vi "Convex Polygon Intersection.vi"(8 "Y 2":dbl[](array[numeric]), 9 "X 2":dbl[](array[numeric]), 10 "Y 1":dbl[](array[numeric]), 11 "X 1":dbl[](array[numeric])) -> (0 "error":i32, 2 "Intersection Y":dbl[](array[numeric]), 3 "Intersection X":dbl[](array[numeric]))   [LabVIEW 2020, in "NI_AAL_Geometry.lvlib"]
doc: "Computes the intersection of two convex polygons."
uses:
  <vilib>/Analysis/NI_AAL_Geometry.lvlib
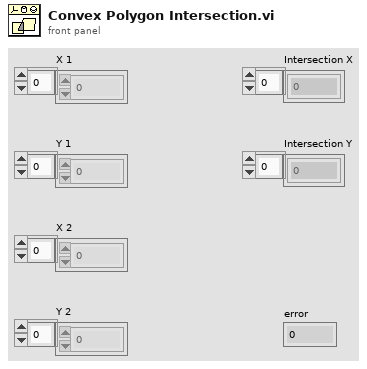
[diagram p1: front panel]
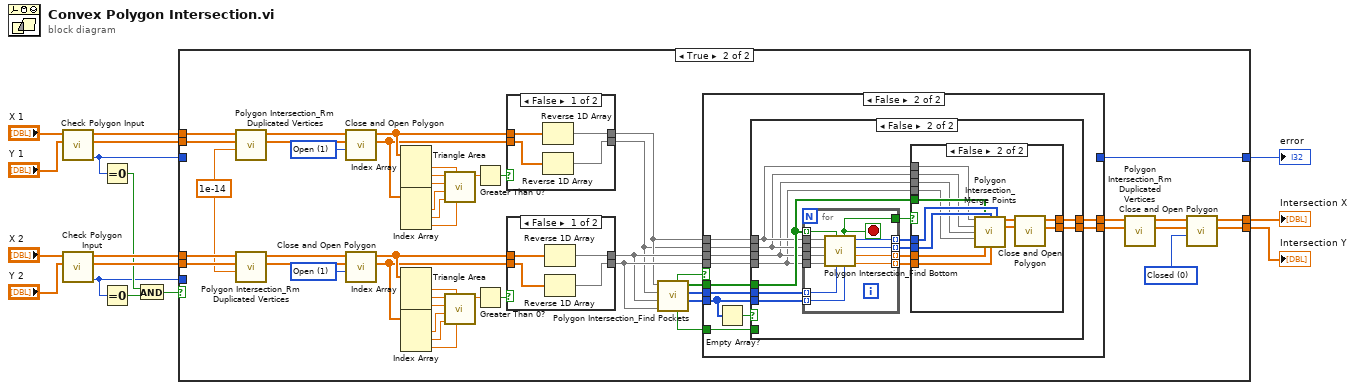
[diagram p0: block diagram]
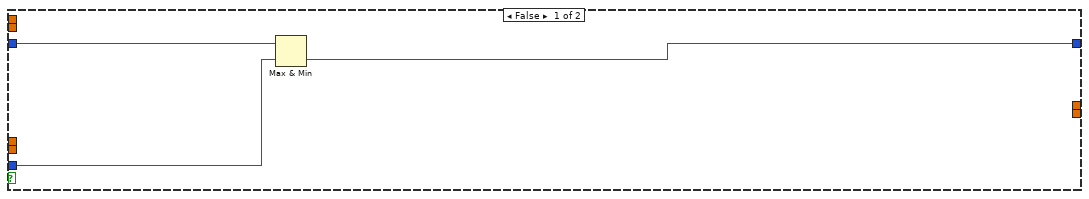
[diagram p2: hidden frame]
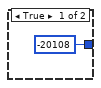
[diagram p3: hidden frame]
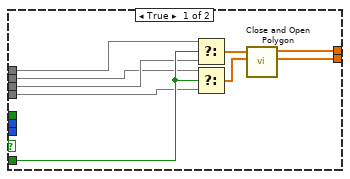
[diagram p4: hidden frame]
diagram:
  n1 = call <vilib>:"Check Polygon Input.vi"("Y In"="Y 1", "X In"="X 1") -> ("error"=w5:i32, "Y Out"=w12:dbl[], "X Out"=w13:dbl[])  [unwired: 7 in]
  n2 = call <vilib>:"Check Polygon Input.vi"("Y In"="Y 2", "X In"="X 2") -> ("error"=w4:i32, "Y Out"=w9:dbl[], "X Out"=w11:dbl[])  [unwired: 7 in]
  n3 = Equal To 0?(x=w5) -> (x = 0?=w8:bool)
  n4 = Equal To 0?(x=w4) -> (x = 0?=w7:bool)
  n5 = And(x=w8, y=w7) -> (x .and. y?=w6:bool)
  n6 = case shown="True" w6 {
    tunnel: w13 -> [_ w28]
    tunnel: w12 -> [_ w27]
    tunnel: w11 -> [_ w24]
    tunnel: w9 -> [_ w23]
    tunnel: w5 -> [w19 _]
    tunnel: w4 -> [w18 _]
    tunnel: [_ w30] -> w3
    tunnel: [w17 w50] -> w2
    tunnel: [_ w29] -> w1
    frame False {
      n7 = Max & Min(x=w19, y=w18) -> (min(x,y)=w17:i32)  [unwired: 1 out]
    }
    frame True {
      w20 = 1e-14 ("tolerance")
      w33 = u16 0 items=["Closed", "Open"] ("type")
      w64 = u16 1 items=["Closed", "Open"] ("type")
      w65 = u16 1 items=["Closed", "Open"] ("type")
      n8 = call <vilib>:"Polygon Intersection_Rm Duplicated Vertices.vi"("tolerance"=w20, "Y"=w27, "X"=w28) -> ("Y out"=w26:dbl[], "X out"=w25:dbl[])  [unwired: 7 in]
      n9 = call <vilib>:"Polygon Intersection_Rm Duplicated Vertices.vi"("tolerance"=w20, "Y"=w23, "X"=w24) -> ("Y out"=w22:dbl[], "X out"=w21:dbl[])  [unwired: 7 in]
      n10 = call <vilib>:"Close and Open Polygon.vi"("type"=w65, "Y In"=w26, "X In"=w25) -> ("Y Out"=w62:dbl[], "X Out"=w63:dbl[])  [unwired: 7 in]
      n11 = call <vilib>:"Close and Open Polygon.vi"("type"=w64, "Y In"=w22, "X In"=w21) -> ("Y Out"=w56:dbl[], "X Out"=w61:dbl[])  [unwired: 7 in]
      n12 = Index Array(array=w63) -> (element #1=w49:dbl, element #2=w48:dbl, element #3=w47:dbl)  [unwired: 3 in]
      n13 = Index Array(array=w62) -> (element #1=w46:dbl, element #2=w45:dbl, element #3=w44:dbl)  [unwired: 3 in]
      n14 = Index Array(array=w61) -> (element #1=w43:dbl, element #2=w42:dbl, element #3=w41:dbl)  [unwired: 3 in]
      n15 = Index Array(array=w56) -> (element #1=w40:dbl, element #2=w39:dbl, element #3=w38:dbl)  [unwired: 3 in]
      n16 = call <vilib>:"Triangle Area.vi"("y 3"=w44, "x 1"=w49, "y 2"=w45, "y 1"=w46, "x 3"=w47, "x 2"=w48) -> ("area"=w37:dbl)  [unwired: 5 in]
      n17 = call <vilib>:"Triangle Area.vi"("y 3"=w38, "x 1"=w43, "y 2"=w39, "y 1"=w40, "x 3"=w41, "x 2"=w42) -> ("area"=w35:dbl)  [unwired: 5 in]
      n18 = Greater Than 0?(x=w37) -> (x > 0?=w36:bool)
      n19 = Greater Than 0?(x=w35) -> (x > 0?=w34:bool)
      n20 = case shown="False" w36 {
        tunnel: w62 -> [w135 w138]
        tunnel: w63 -> [w137 w139]
        tunnel: [w136 w139] -> w52
        tunnel: [w134 w138] -> w51
        frame False {
          n21 = Reverse 1D Array(array=w137) -> (reversed array=w136:dbl[])
          n22 = Reverse 1D Array(array=w135) -> (reversed array=w134:dbl[])
        }
        frame True {
        }
      }
      n23 = case shown="False" w34 {
        tunnel: w56 -> [w129 w132]
        tunnel: w61 -> [w131 w133]
        tunnel: [w130 w133] -> w57
        tunnel: [w128 w132] -> w60
        frame False {
          n24 = Reverse 1D Array(array=w131) -> (reversed array=w130:dbl[])
          n25 = Reverse 1D Array(array=w129) -> (reversed array=w128:dbl[])
        }
        frame True {
        }
      }
      n26 = call <vilib>:"Polygon Intersection_Find Pockets.vi"("y2"=w60, "x2"=w57, "y1"=w51, "x1"=w52) -> ("index2"=w59:i32[], "index1"=w67:i32[], "left turn?"=w66:bool[], "inner?"=w58:bool, "complex or concave?"=w53:bool)  [unwired: 3 in]
      n27 = case shown="False" w53 {
        tunnel: w67 -> [_ w79]
        tunnel: w59 -> [_ w71]
        tunnel: w66 -> [_ w78]
        tunnel: [_ w77] -> w55
        tunnel: w52 -> [_ w76]
        tunnel: w51 -> [_ w75]
        tunnel: w57 -> [_ w74]
        tunnel: w60 -> [_ w73]
        tunnel: [_ w72] -> w54
        tunnel: w58 -> [_ w69]
        tunnel: [-20108 _] -> w50
        frame True {
        }
        frame False {
          n28 = Empty Array?(array=w71) -> (empty?=w70:bool)
          n29 = case shown="False" w70 {
            tunnel: w79 -> [_ w102]
            tunnel: w71 -> [_ w101]
            tunnel: w78 -> [_ w93]
            tunnel: [w81 w96] -> w77
            tunnel: [w80 w95] -> w72
            tunnel: w76 -> [w88 w92]
            tunnel: w75 -> [w85 w91]
            tunnel: w74 -> [w86 w90]
            tunnel: w73 -> [w84 w89]
            tunnel: w69 -> [w87 _]
            frame True {
              n30 = Select(t=w88, s=w87, f=w86) -> (s? t:f=w83:dbl[])
              n31 = Select(t=w85, s=w87, f=w84) -> (s? t:f=w82:dbl[])
              n32 = call <vilib>:"Close and Open Polygon.vi"("Y In"=w82, "X In"=w83) -> ("Y Out"=w80:dbl[], "X Out"=w81:dbl[])  [unwired: 8 in]
            }
            frame False {
              n33 = for {
                tunnel: w92 -> [w124]
                tunnel: w91 -> [w123]
                tunnel: w90 -> [w122]
                tunnel: w89 -> [w121]
                tunnel: w93 -> [w125] mode=indexing
                tunnel: w102 -> [w127] mode=indexing
                tunnel: w101 -> [w126] mode=indexing
                tunnel: [w118] -> w100 mode=indexing
                tunnel: [w117] -> w99 mode=indexing
                tunnel: [w120] -> w98 mode=indexing
                tunnel: [w119] -> w97 mode=indexing
                tunnel: [w116] -> w94
                stop <- w116 stop-if-true
                n34 = call <vilib>:"Polygon Intersection_Find Bottom.vi"("index2"=w126, "index1"=w127, "Left Turn?"=w125, "y2"=w121, "x2"=w122, "y1"=w123, "x1"=w124) -> ("y"=w119:dbl, "x"=w120:dbl, "index2 out"=w117:i32, "index1 out"=w118:i32, "isolate?"=w116:bool)
              }
              n35 = case shown="False" w94 {
                tunnel: w100 -> [_ w115]
                tunnel: w99 -> [_ w114]
                tunnel: w93 -> [_ w113]
                tunnel: w98 -> [_ w112]
                tunnel: w97 -> [_ w111]
                tunnel: [_ w104] -> w96
                tunnel: [_ w103] -> w95
                tunnel: w90 -> [_ w110]
                tunnel: w89 -> [_ w109]
                tunnel: w92 -> [_ w108]
                tunnel: w91 -> [_ w107]
                frame True {
                }
                frame False {
                  n36 = call <vilib>:"Polygon Intersection_Merge Points.vi"("x1"=w108, "left turn?"=w113, "index2"=w114, "index1"=w115, "y1"=w107, "x2"=w110, "y2"=w109, "xi"=w112, "yi"=w111) -> ("x"=w106:dbl[], "y"=w105:dbl[])  [unwired: 5 in]
                  n37 = call <vilib>:"Close and Open Polygon.vi"("Y In"=w105, "X In"=w106) -> ("Y Out"=w103:dbl[], "X Out"=w104:dbl[])  [unwired: 8 in]
                }
              }
            }
          }
        }
      }
      n38 = call <vilib>:"Polygon Intersection_Rm Duplicated Vertices.vi"("Y"=w54, "X"=w55) -> ("Y out"=w32:dbl[], "X out"=w31:dbl[])  [unwired: 8 in]
      n39 = call <vilib>:"Close and Open Polygon.vi"("type"=w33, "Y In"=w32, "X In"=w31) -> ("Y Out"=w29:dbl[], "X Out"=w30:dbl[])  [unwired: 7 in]
    }
  }
  "Intersection X" <- w3
  "Intersection Y" <- w1
  "error" <- w2
